vi "Remove All Devices.vi"(8 "error in (no error)":errorcluster, 11 "Controller in":refnum<class "Controller.lvclass">) -> (0 "error out":errorcluster, 3 "Controller out":refnum<class "Controller.lvclass">)   [LabVIEW 2016, in "Controller Actor.lvlib" / "Controller.lvclass"]
uses:
  <userlib>/Common Components/Controller/Controller.lvclass
  <userlib>/Common Components/Controller/Controller.lvclass/Controller.ctl
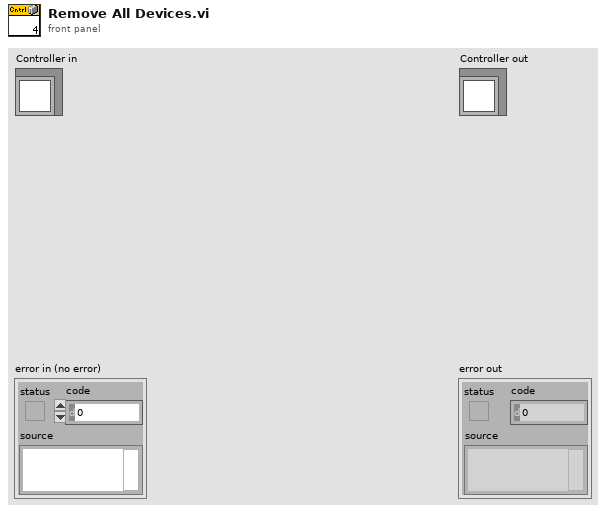
[diagram p1: front panel]
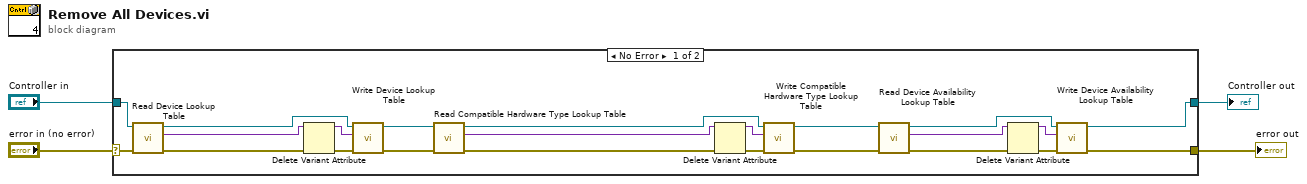
[diagram p0: block diagram]
diagram:
  n1 = case shown="No Error" "error in (no error)" {
    selector: "error in (no error)" -> [w26 w29]
    tunnel: [w17 w29] -> w1
    tunnel: [w20 w28] -> w2
    tunnel: "Controller in" -> [w27 w28]
    frame No Error {
      n2 = call <userlib>:"Read Device Lookup Table.vi"("error in (no error)"=w26, "Controller in"=w27) -> ("error out"=w10:errorcluster, "Device Lookup Table (Device GUID -> Device Object)"=w16:variant, "Controller out"=w25:refnum<class "Controller.lvclass">)  [unwired: 7 in]
      n3 = Delete Variant Attribute(4:w10, 7:w16) -> (0:w9:errorcluster, 3:w15:variant)  [unwired: 1 in, 1 out]
      n4 = call <userlib>:"Write Device Lookup Table.vi"("error in (no error)"=w9, "Device Lookup Table (Device GUID -> Device Object)"=w15, "Controller in"=w25) -> ("error out"=w19:errorcluster, "Controller out"=w24:refnum<class "Controller.lvclass">)  [unwired: 7 in]
      n5 = call <userlib>:"Read Compatible Hardware Type Lookup Table.vi"("error in (no error)"=w19, "Controller in"=w24) -> ("error out"=w8:errorcluster, "Compatible Hardware Type Lookup Table"=w14:variant, "Controller out"=w23:refnum<class "Controller.lvclass">)  [unwired: 7 in]
      n6 = Delete Variant Attribute(4:w8, 7:w14) -> (0:w7:errorcluster, 3:w13:variant)  [unwired: 1 in, 1 out]
      n7 = call <userlib>:"Write Compatible Hardware Type Lookup Table.vi"("error in (no error)"=w7, "Compatible Hardware Type Lookup Table"=w13, "Controller in"=w23) -> ("error out"=w18:errorcluster, "Controller out"=w22:refnum<class "Controller.lvclass">)  [unwired: 7 in]
      n8 = call <userlib>:"Read Device Availability Lookup Table.vi"("error in (no error)"=w18, "Controller in"=w22) -> ("error out"=w6:errorcluster, "Device Availability Lookup Table"=w12:variant, "Controller out"=w21:refnum<class "Controller.lvclass">)  [unwired: 7 in]
      n9 = Delete Variant Attribute(4:w6, 7:w12) -> (0:w5:errorcluster, 3:w11:variant)  [unwired: 1 in, 1 out]
      n10 = call <userlib>:"Write Device Availability Lookup Table.vi"("error in (no error)"=w5, "Device Availability Lookup Table"=w11, "Controller in"=w21) -> ("error out"=w17:errorcluster, "Controller out"=w20:refnum<class "Controller.lvclass">)  [unwired: 7 in]
    }
    frame Error {
    }
  }
  "error out" <- w1
  "Controller out" <- w2
